vi "Select_Value_backup.vi"(2 "Numerisch":i32, 3 "System Monitor Variables":T1) -> (0 "Array":dbl[](array[numeric]), 1 "Value":dbl format="%#_13g")   [LabVIEW 2016]
uses:
  Global/Global Variables/System Monitor Cluster.ctl
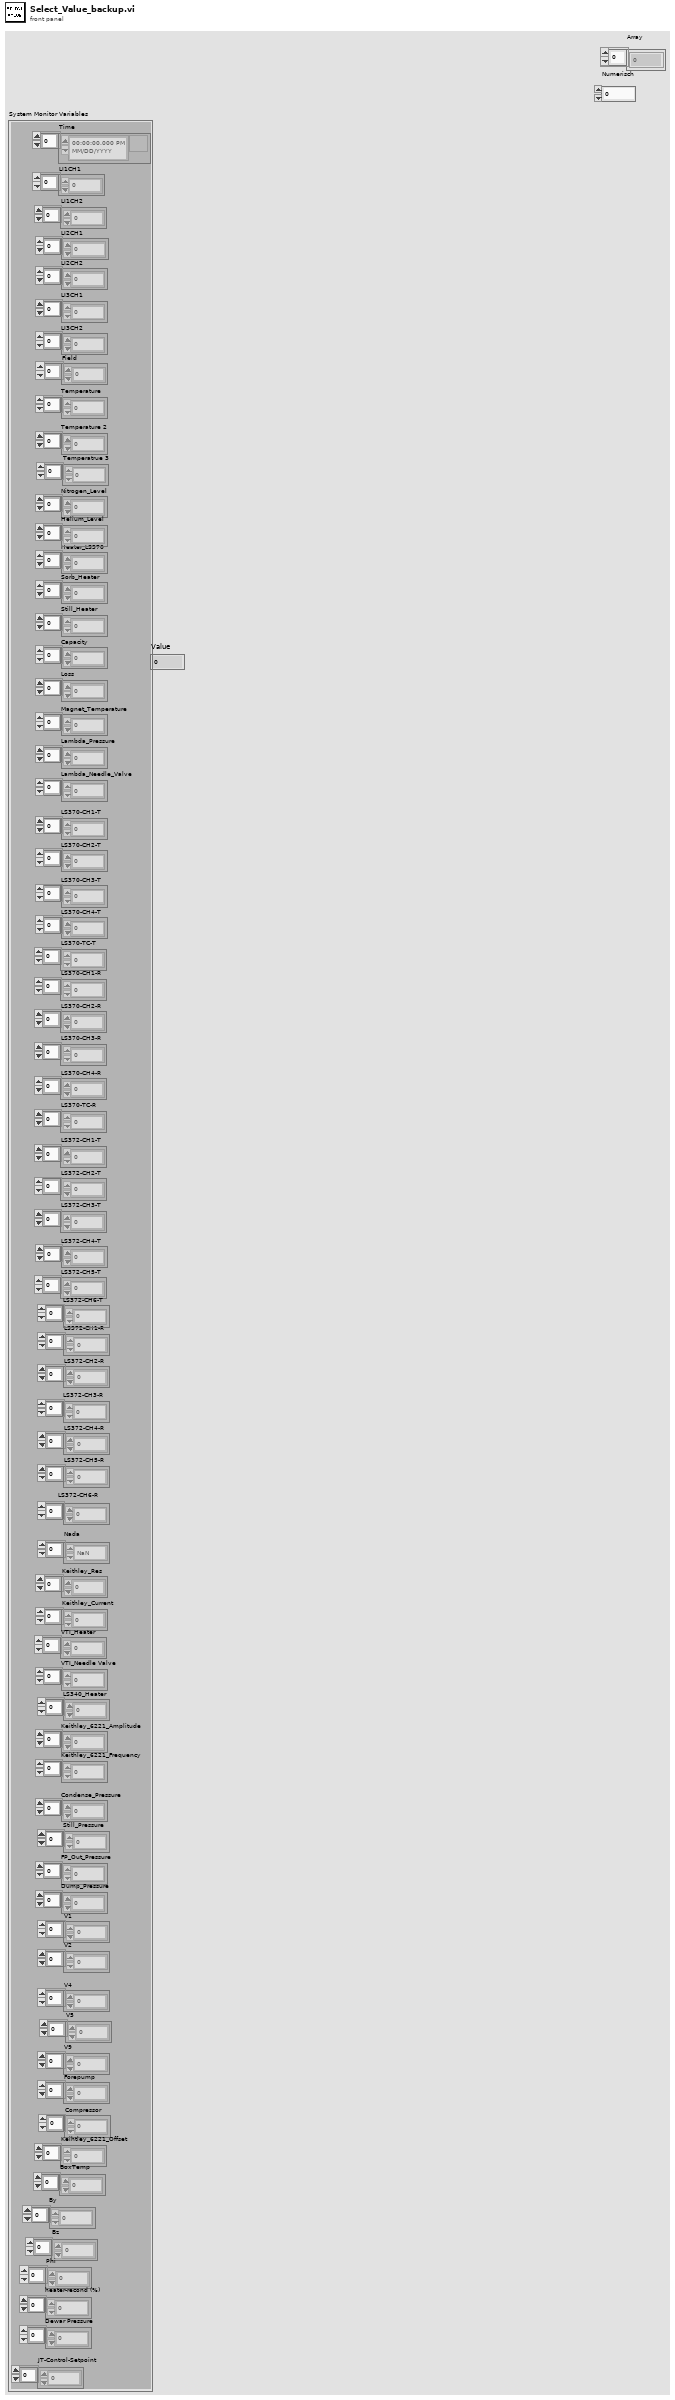
[diagram p1: front panel]
types:
  T1 = typedef "System Monitor Cluster.ctl" = cluster{"Time":timestamp[], "LI1CH1":dbl[], "LI1CH2":dbl[], "LI2CH1":dbl[], "LI2CH2":dbl[], "LI3CH1":dbl[], "LI3CH2":dbl[], "Field":dbl[], "Temperature":dbl[], "Temperature 2":dbl[], "Temperatrue 3":dbl[], "Nitrogen_Level":dbl[], "Helium_Level":dbl[], "Heater_LS370":dbl[], "Sorb_Heater":dbl[], "Still_Heater":dbl[], "Capacity":dbl[], "Loss":dbl[], "Magnet_Temperature":dbl[], "Lambda_Pressure":dbl[], "Lambda_Needle_Valve":dbl[], "LS370-CH1-T":dbl[], "LS370-CH2-T":dbl[], "LS370-CH3-T":dbl[], "LS370-CH4-T":dbl[], "LS370-TC-T":dbl[], "LS370-CH1-R":dbl[], "LS370-CH2-R":dbl[], "LS370-CH3-R":dbl[], "LS370-CH4-R":dbl[], "LS370-TC-R":dbl[], "LS372-CH1-T":dbl[], "LS372-CH2-T":dbl[], "LS372-CH3-T":dbl[], "LS372-CH4-T":dbl[], "LS372-CH5-T":dbl[], "LS372-CH6-T":dbl[], "LS372-CH1-R":dbl[], "LS372-CH2-R":dbl[], "LS372-CH3-R":dbl[], "LS372-CH4-R":dbl[], "LS372-CH5-R":dbl[], "LS372-CH6-R":dbl[], "Nada":dbl[], "Keithley_Res":dbl[], "Keithley_Current":dbl[], "VTI_Heater":dbl[], "VTI_Needle Valve":dbl[], "LS340_Heater":dbl[], "Keithley_6221_Amplitude":dbl[], "Keithley_6221_Frequency":dbl[], "Condense_Pressure":dbl[], "Still_Pressure":dbl[], "FP_Out_Pressure":dbl[], "Dump_Pressure":dbl[], "V1":dbl[], "V2":dbl[], "V4":dbl[], "V5":dbl[], "V9":dbl[], "Forepump":dbl[], "Compressor":dbl[], "Keihtley_6221_Offset":dbl[], "BoxTemp":dbl[], "By":dbl[], "Bz":dbl[], "Phi":dbl[], "heater-recond (%)":dbl[], "Dewar Pressure ":dbl[], "JT-Control-Setpoint":dbl[]}
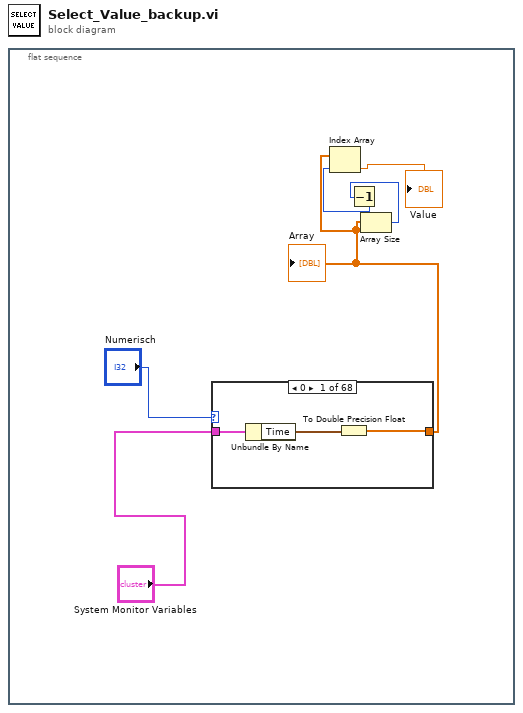
[diagram p0: block diagram]
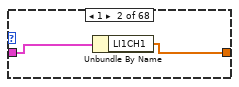
[diagram p2: hidden frame]
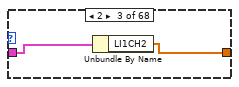
[diagram p3: hidden frame]
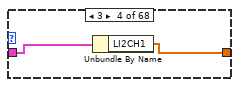
[diagram p4: hidden frame]
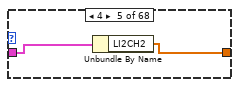
[diagram p5: hidden frame]
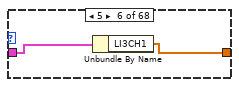
[diagram p6: hidden frame]
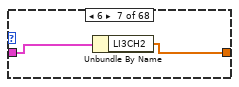
[diagram p7: hidden frame]
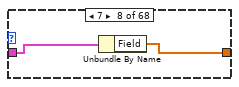
[diagram p8: hidden frame]
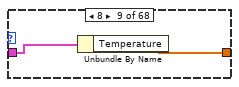
[diagram p9: hidden frame]
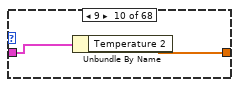
[diagram p10: hidden frame]
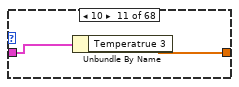
[diagram p11: hidden frame]
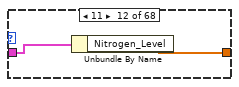
[diagram p12: hidden frame]
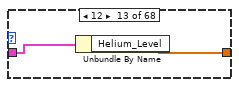
[diagram p13: hidden frame]
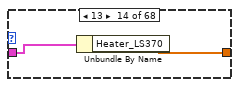
[diagram p14: hidden frame]
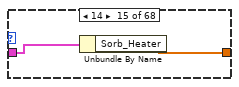
[diagram p15: hidden frame]
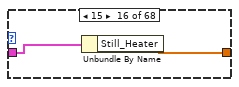
[diagram p16: hidden frame]
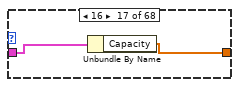
[diagram p17: hidden frame]
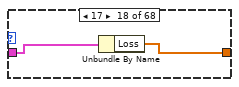
[diagram p18: hidden frame]
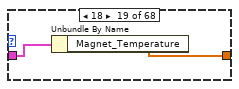
[diagram p19: hidden frame]
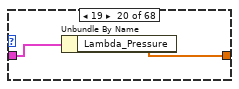
[diagram p20: hidden frame]
diagram:
  n1 = flat-sequence {
    frame #0 {
      n2 = case shown="0" "Numerisch" {
        tunnel: "System Monitor Variables" -> [w9 w11 w13 w15 w17 w19 w21 w23 w25 w27 w29 w31 w33 w35 w37 w39 w41 w43 w45 w47 w49 w51 w53 w55 w57 w59 w61 w63 w65 w67 w69 w71 w73 w75 w77 w79 w81 w83 w85 w87 w89 w91 w93 w95 w97 w99 w101 w103 w105 w107 w109 w111 w113 w115 w117 w119 w121 w123 w125 w127 w129 w131 w133 w135 w137 w139 w141 w143]
        tunnel: [w7 w10 w12 w14 w16 w18 w20 w22 w24 w26 w28 w30 w32 w34 w36 w38 w40 w42 w44 w46 w48 w50 w52 w54 w56 w58 w60 w62 w64 w66 w68 w70 w72 w74 w76 w78 w80 w82 w84 w86 w88 w90 w92 w94 w96 w98 w100 w102 w104 w106 w108 w110 w112 w114 w116 w118 w120 w122 w124 w126 w128 w130 w132 w134 w136 w138 w140 w142] -> w4
        frame 0 {
          n3 = Unbundle By Name(w9) -> ("Time"=w8:timestamp[])
          n4 = To Double Precision Float(number=w8) -> (double precision float=w7:dbl[])
        }
        frame 1 {
          n5 = Unbundle By Name(w11) -> ("LI1CH1"=w10:dbl[])
        }
        frame 2 {
          n6 = Unbundle By Name(w13) -> ("LI1CH2"=w12:dbl[])
        }
        frame 3 {
          n7 = Unbundle By Name(w15) -> ("LI2CH1"=w14:dbl[])
        }
        frame 4 {
          n8 = Unbundle By Name(w17) -> ("LI2CH2"=w16:dbl[])
        }
        frame 5 {
          n9 = Unbundle By Name(w19) -> ("LI3CH1"=w18:dbl[])
        }
        frame 6 {
          n10 = Unbundle By Name(w21) -> ("LI3CH2"=w20:dbl[])
        }
        frame 7 {
          n11 = Unbundle By Name(w23) -> ("Field"=w22:dbl[])
        }
        frame 8 {
          n12 = Unbundle By Name(w25) -> ("Temperature"=w24:dbl[])
        }
        frame 9 {
          n13 = Unbundle By Name(w27) -> ("Temperature 2"=w26:dbl[])
        }
        frame 10 {
          n14 = Unbundle By Name(w29) -> ("Temperatrue 3"=w28:dbl[])
        }
        frame 11 {
          n15 = Unbundle By Name(w31) -> ("Nitrogen_Level"=w30:dbl[])
        }
        frame 12 {
          n16 = Unbundle By Name(w33) -> ("Helium_Level"=w32:dbl[])
        }
        frame 13 {
          n17 = Unbundle By Name(w35) -> ("Heater_LS370"=w34:dbl[])
        }
        frame 14 {
          n18 = Unbundle By Name(w37) -> ("Sorb_Heater"=w36:dbl[])
        }
        frame 15 {
          n19 = Unbundle By Name(w39) -> ("Still_Heater"=w38:dbl[])
        }
        frame 16 {
          n20 = Unbundle By Name(w41) -> ("Capacity"=w40:dbl[])
        }
        frame 17 {
          n21 = Unbundle By Name(w43) -> ("Loss"=w42:dbl[])
        }
        frame 18 {
          n22 = Unbundle By Name(w45) -> ("Magnet_Temperature"=w44:dbl[])
        }
        frame 19 {
          n23 = Unbundle By Name(w47) -> ("Lambda_Pressure"=w46:dbl[])
        }
        frame 20 {
          n24 = Unbundle By Name(w49) -> ("Lambda_Needle_Valve"=w48:dbl[])
        }
        frame 21 {
          n25 = Unbundle By Name(w51) -> ("LS370-CH1-T"=w50:dbl[])
        }
        frame 22 {
          n26 = Unbundle By Name(w53) -> ("LS370-CH2-T"=w52:dbl[])
        }
        frame 23 {
          n27 = Unbundle By Name(w55) -> ("LS370-CH3-T"=w54:dbl[])
        }
        frame 24 {
          n28 = Unbundle By Name(w57) -> ("LS370-CH4-T"=w56:dbl[])
        }
        frame 25 {
          n29 = Unbundle By Name(w59) -> ("LS370-TC-T"=w58:dbl[])
        }
        frame 26 {
          n30 = Unbundle By Name(w61) -> ("LS370-CH1-R"=w60:dbl[])
        }
        frame 27 {
          n31 = Unbundle By Name(w63) -> ("LS370-CH2-R"=w62:dbl[])
        }
        frame 28 {
          n32 = Unbundle By Name(w65) -> ("LS370-CH3-R"=w64:dbl[])
        }
        frame 29 {
          n33 = Unbundle By Name(w67) -> ("LS370-CH4-R"=w66:dbl[])
        }
        frame 30 {
          n34 = Unbundle By Name(w69) -> ("LS370-TC-R"=w68:dbl[])
        }
        frame 31 {
          n35 = Unbundle By Name(w71) -> ("LS372-CH1-T"=w70:dbl[])
        }
        frame 32 {
          n36 = Unbundle By Name(w73) -> ("LS372-CH2-T"=w72:dbl[])
        }
        frame 33 {
          n37 = Unbundle By Name(w75) -> ("LS372-CH3-T"=w74:dbl[])
        }
        frame 34 {
          n38 = Unbundle By Name(w77) -> ("LS372-CH4-T"=w76:dbl[])
        }
        frame 35 {
          n39 = Unbundle By Name(w79) -> ("LS372-CH5-T"=w78:dbl[])
        }
        frame 36 {
          n40 = Unbundle By Name(w81) -> ("LS372-CH1-R"=w80:dbl[])
        }
        frame 37 {
          n41 = Unbundle By Name(w83) -> ("LS372-CH2-R"=w82:dbl[])
        }
        frame 38 {
          n42 = Unbundle By Name(w85) -> ("LS372-CH3-R"=w84:dbl[])
        }
        frame 39 {
          n43 = Unbundle By Name(w87) -> ("LS372-CH4-R"=w86:dbl[])
        }
        frame 40 {
          n44 = Unbundle By Name(w89) -> ("LS372-CH5-R"=w88:dbl[])
        }
        frame 41, Default {
          n45 = Unbundle By Name(w91) -> ("Nada"=w90:dbl[])
        }
        frame 42 {
          n46 = Unbundle By Name(w93) -> ("Keithley_Res"=w92:dbl[])
        }
        frame 43 {
          n47 = Unbundle By Name(w95) -> ("Keithley_Current"=w94:dbl[])
        }
        frame 44 {
          n48 = Unbundle By Name(w97) -> ("VTI_Heater"=w96:dbl[])
        }
        frame 45 {
          n49 = Unbundle By Name(w99) -> ("VTI_Needle Valve"=w98:dbl[])
        }
        frame 46 {
          n50 = Unbundle By Name(w101) -> ("LS340_Heater"=w100:dbl[])
        }
        frame 47 {
          n51 = Unbundle By Name(w103) -> ("Keithley_6221_Amplitude"=w102:dbl[])
        }
        frame 48 {
          n52 = Unbundle By Name(w105) -> ("Keithley_6221_Frequency"=w104:dbl[])
        }
        frame 49 {
          n53 = Unbundle By Name(w107) -> ("Condense_Pressure"=w106:dbl[])
        }
        frame 50 {
          n54 = Unbundle By Name(w109) -> ("Still_Pressure"=w108:dbl[])
        }
        frame 51 {
          n55 = Unbundle By Name(w111) -> ("FP_Out_Pressure"=w110:dbl[])
        }
        frame 52 {
          n56 = Unbundle By Name(w113) -> ("Dump_Pressure"=w112:dbl[])
        }
        frame 53 {
          n57 = Unbundle By Name(w115) -> ("V1"=w114:dbl[])
        }
        frame 54 {
          n58 = Unbundle By Name(w117) -> ("V2"=w116:dbl[])
        }
        frame 55 {
          n59 = Unbundle By Name(w119) -> ("V4"=w118:dbl[])
        }
        frame 56 {
          n60 = Unbundle By Name(w121) -> ("V5"=w120:dbl[])
        }
        frame 57 {
          n61 = Unbundle By Name(w123) -> ("V9"=w122:dbl[])
        }
        frame 58 {
          n62 = Unbundle By Name(w125) -> ("Forepump"=w124:dbl[])
        }
        frame 59 {
          n63 = Unbundle By Name(w127) -> ("Compressor"=w126:dbl[])
        }
        frame 60 {
          n64 = Unbundle By Name(w129) -> ("Keihtley_6221_Offset"=w128:dbl[])
        }
        frame 61 {
          n65 = Unbundle By Name(w131) -> ("BoxTemp"=w130:dbl[])
        }
        frame 62 {
          n66 = Unbundle By Name(w133) -> ("By"=w132:dbl[])
        }
        frame 63 {
          n67 = Unbundle By Name(w135) -> ("Bz"=w134:dbl[])
        }
        frame 64 {
          n68 = Unbundle By Name(w137) -> ("Phi"=w136:dbl[])
        }
        frame 65 {
          n69 = Unbundle By Name(w139) -> ("heater-recond (%)"=w138:dbl[])
        }
        frame 66 {
          n70 = Unbundle By Name(w141) -> ("Dewar Pressure"=w140:dbl[])
        }
        frame 67 {
          n71 = Unbundle By Name(w143) -> ("JT-Control-Setpoint"=w142:dbl[])
        }
      }
      "Array" <- w4
      n72 = Array Size(array=w4) -> (size(s)=w2:i32)
      n73 = Decrement(x=w2) -> (x-1=w1:i32)
      n74 = Index Array(array=w4, index=w1) -> (element=→"Value":dbl)
    }
  }
